vi "ReadParameter.vi"(0 "ParameterConf in":refnum<class "ParameterConf.lvclass">, 3 "error in (no error)":errorcluster, 4 "Parameter":T3(ring)) -> (7 "ParameterConf out":refnum<class "ParameterConf.lvclass">, 8 "DataOut":variant, 9 "DataOutClust":T2, 10 "error out":errorcluster)   [LabVIEW 2014, in "LibraryGcode.lvlib" / "ParameterConf.lvclass"]
uses:
  ParameterConf.lvclass
  control/TypeFirmwareControl.ctl
  ParameterConf.lvclass/ParameterConf.ctl
  LibraryGcode.lvlib
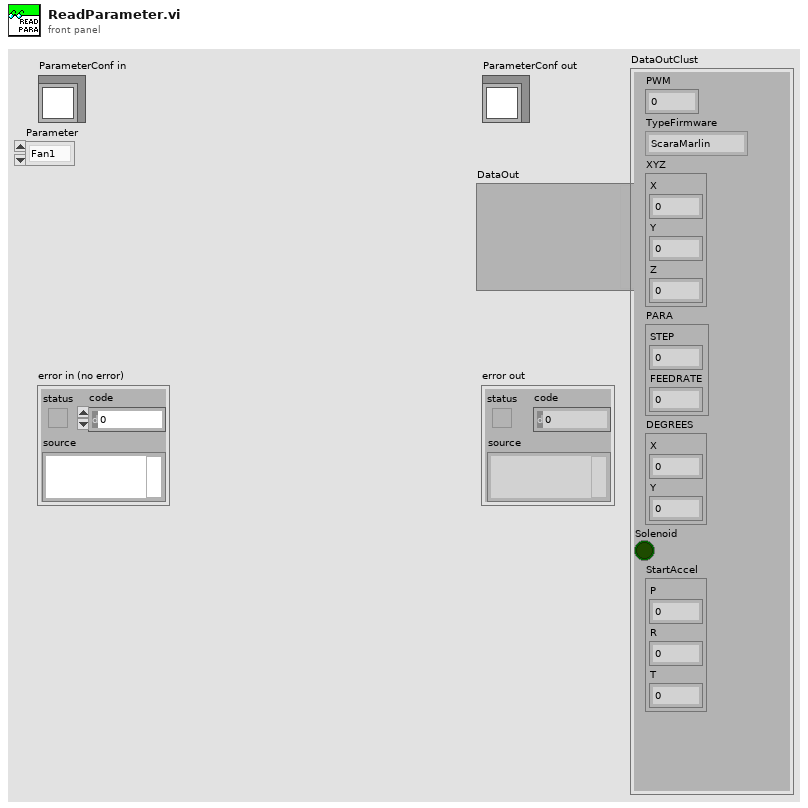
[diagram p1: front panel]
types:
  T1 = typedef "LibraryGcode.lvlib/TypeFirmwareControl.ctl" = enum16{"ScaraMarlin", "CncMarlin", "Mk4Due"}
  T2 = cluster{"PWM":dbl, "TypeFirmware":T1, "XYZ":cluster{"X":dbl, "Y":dbl, "Z":dbl}, "PARA":cluster{"STEP":i16, "FEEDRATE":dbl}, "DEGREES":cluster{"X":dbl, "Y":dbl}, "Solenoid":bool, "StartAccel":cluster{"P":dbl, "R":dbl, "T":dbl}}
  T3 = enum16{"Fan1", "Fan2", "Fan3", "PARA", "POS_DEGREE", "Solenoid", "Spindle", "TypeFirmware", "WaitPin", "MaxAcel", "MaxFeedrate", "MaxSize", "MaxStartAccel"}
  T4 = cluster{"POS":cluster{"X":dbl, "Y":dbl, "Z":dbl}, "DEGREES":cluster{"X":dbl, "Y":dbl}}
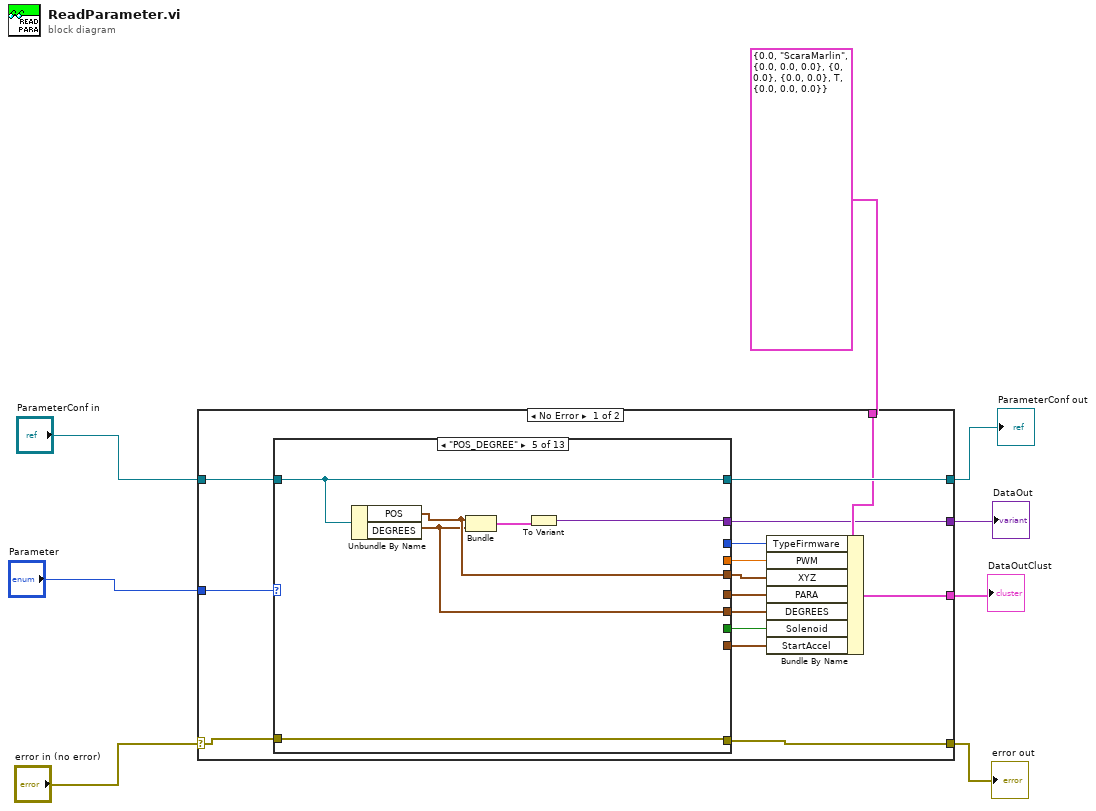
[diagram p0: block diagram]
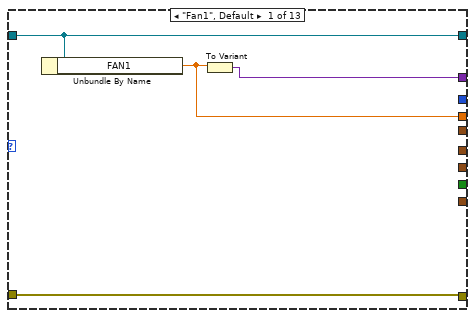
[diagram p2: hidden frame]
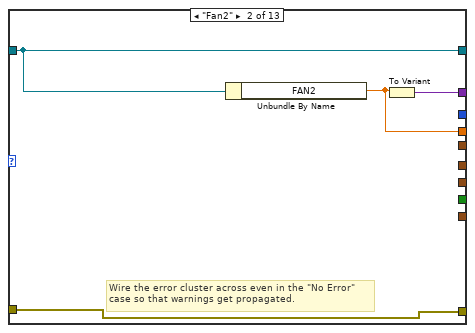
[diagram p3: hidden frame]
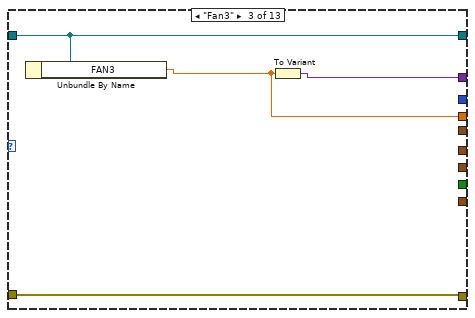
[diagram p4: hidden frame]
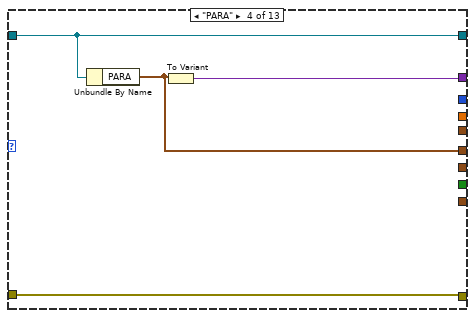
[diagram p5: hidden frame]
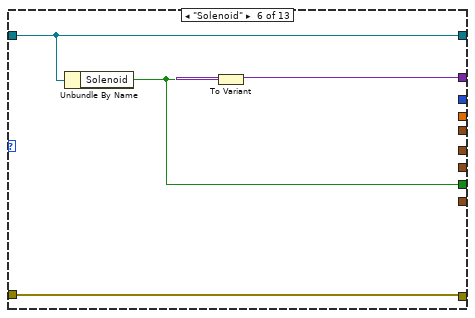
[diagram p6: hidden frame]
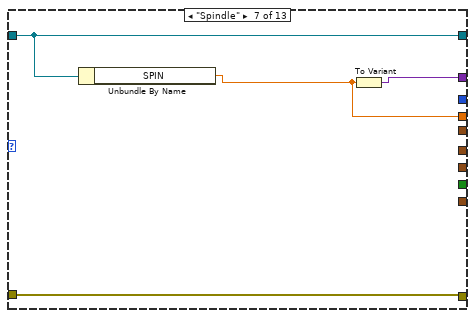
[diagram p7: hidden frame]
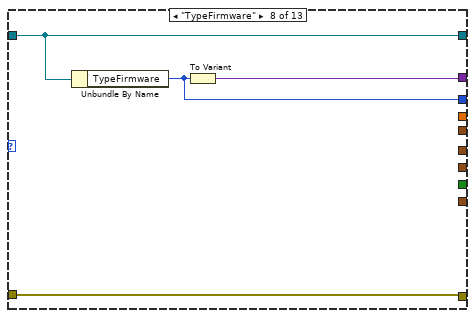
[diagram p8: hidden frame]
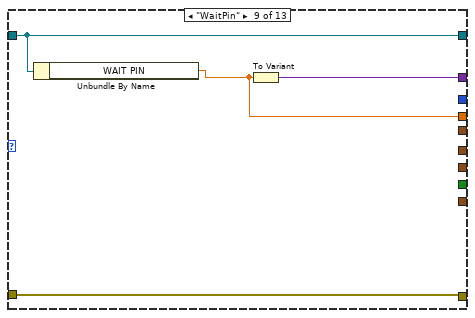
[diagram p9: hidden frame]
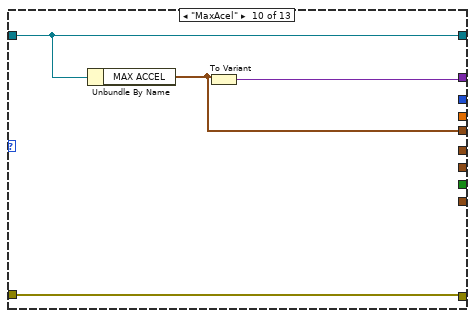
[diagram p10: hidden frame]
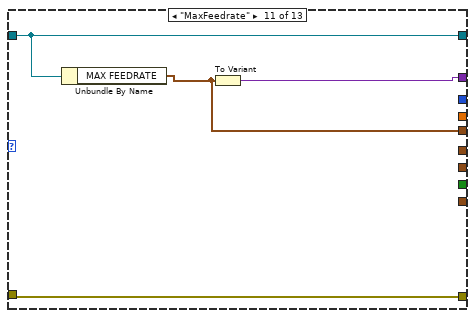
[diagram p11: hidden frame]
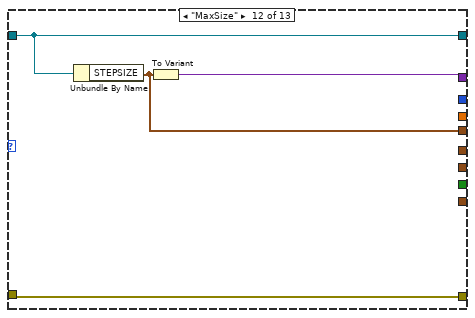
[diagram p12: hidden frame]
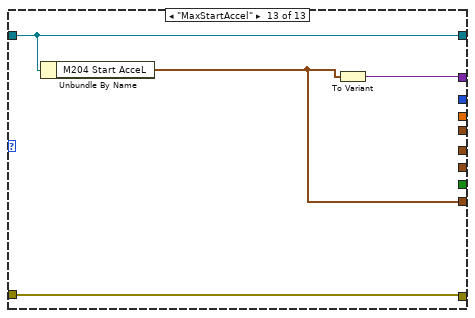
[diagram p13: hidden frame]
diagram:
  n1 = case shown="No Error" "error in (no error)" {
    selector: "error in (no error)" -> [w20 w79]
    tunnel: [w21 w79] -> w7
    tunnel: [w23 w78] -> w5
    tunnel: "ParameterConf in" -> [w22 w78]
    tunnel: "Parameter" -> [w19 _]
    tunnel: [w16 _] -> w3
    tunnel: T2 {"PWM"=0.0, "TypeFirmware"=enum."ScaraMarlin", "XYZ"={"X"=0.0, "Y"=0.0, "Z"=0.0}, "PARA"={"STEP"=0, "FEEDRATE"=0.0}, "DEGREES"={"X"=0.0, "Y"=0.0}, "Solenoid"=TRUE, "StartAccel"={"P"=0.0, "R"=0.0, "T"=0.0}} ("input cluster") -> [w18 _]
    tunnel: [w9 _] -> w1
    frame No Error {
      n2 = case shown="\"POS_DEGREE\"" w19 {
        tunnel: [w27 w30 w35 w39 w45 w49 w53 w57 w60 w64 w69 w73 w76] -> w23
        tunnel: w22 -> [w27 w30 w35 w39 w45 w49 w53 w57 w60 w64 w69 w73 w76]
        tunnel: [w26 w31 w33 w37 w43 w47 w52 w55 w61 w65 w67 w71 w77] -> w21
        tunnel: w20 -> [w26 w31 w33 w37 w43 w47 w52 w55 w61 w65 w67 w71 w77]
        tunnel: [w25 w29 w34 w38 w44 w48 w51 w56 w59 w63 w68 w72 w75] -> w16
        tunnel: [_ _ _ _ w41 _ _ _ _ w62 w66 w70 _] -> w17
        tunnel: [w24 w28 w32 _ _ _ w50 _ w58 _ _ _ _] -> w15
        tunnel: [_ _ _ w36 _ _ _ _ _ _ _ _ _] -> w14
        tunnel: [_ _ _ _ w40 _ _ _ _ _ _ _ _] -> w13
        tunnel: [_ _ _ _ _ w46 _ _ _ _ _ _ _] -> w12
        tunnel: [_ _ _ _ _ _ _ w54 _ _ _ _ _] -> w11
        tunnel: [_ _ _ _ _ _ _ _ _ _ _ _ w74] -> w10
        frame "Fan1", Default {
          n3 = Unbundle By Name(w27) -> ("FAN1"=w24:dbl)
          n4 = To Variant(anything=w24) -> (Variant=w25:variant)
        }
        frame "Fan2" {
          # "Wire the error cluster across even in the \"No Error\"\ncase so that warnings get propagated."
          n5 = Unbundle By Name(w30) -> ("FAN2"=w28:dbl)
          n6 = To Variant(anything=w28) -> (Variant=w29:variant)
        }
        frame "Fan3" {
          n7 = Unbundle By Name(w35) -> ("FAN3"=w32:dbl)
          n8 = To Variant(anything=w32) -> (Variant=w34:variant)
        }
        frame "PARA" {
          n9 = Unbundle By Name(w39) -> ("PARA"=w36:cluster{"STEP":i16, "FEEDRATE":dbl})
          n10 = To Variant(anything=w36) -> (Variant=w38:variant)
        }
        frame "POS_DEGREE" {
          n11 = Unbundle By Name(w45) -> ("POS"=w41:cluster{"X":dbl, "Y":dbl, "Z":dbl}, "DEGREES"=w40:cluster{"X":dbl, "Y":dbl})
          n12 = Bundle("POS"=w41, "DEGREES"=w40) -> (w42:T4)  [unwired: 1 in]
          n13 = To Variant(anything=w42) -> (Variant=w44:variant)
        }
        frame "Solenoid" {
          n14 = Unbundle By Name(w49) -> ("Solenoid"=w46:bool)
          n15 = To Variant(anything=w46) -> (Variant=w48:variant)
        }
        frame "Spindle" {
          n16 = Unbundle By Name(w53) -> ("SPIN"=w50:dbl)
          n17 = To Variant(anything=w50) -> (Variant=w51:variant)
        }
        frame "TypeFirmware" {
          n18 = Unbundle By Name(w57) -> ("TypeFirmware"=w54:T1)
          n19 = To Variant(anything=w54) -> (Variant=w56:variant)
        }
        frame "WaitPin" {
          n20 = Unbundle By Name(w60) -> ("WAIT PIN"=w58:dbl)
          n21 = To Variant(anything=w58) -> (Variant=w59:variant)
        }
        frame "MaxAcel" {
          n22 = Unbundle By Name(w64) -> ("MAX ACCEL"=w62:cluster{"X":dbl, "Y":dbl, "Z":dbl})
          n23 = To Variant(anything=w62) -> (Variant=w63:variant)
        }
        frame "MaxFeedrate" {
          n24 = Unbundle By Name(w69) -> ("MAX FEEDRATE"=w66:cluster{"X":dbl, "Y":dbl, "Z":dbl})
          n25 = To Variant(anything=w66) -> (Variant=w68:variant)
        }
        frame "MaxSize" {
          n26 = Unbundle By Name(w73) -> ("STEPSIZE"=w70:cluster{"X":dbl, "Y":dbl, "Z":dbl})
          n27 = To Variant(anything=w70) -> (Variant=w72:variant)
        }
        frame "MaxStartAccel" {
          n28 = Unbundle By Name(w76) -> ("M204 Start AcceL"=w74:cluster{"P":dbl, "R":dbl, "T":dbl})
          n29 = To Variant(anything=w74) -> (Variant=w75:variant)
        }
      }
      n30 = Bundle By Name(cluster=w18, "TypeFirmware"=w11, "PWM"=w15, "XYZ"=w17, "PARA"=w14, "DEGREES"=w13, "Solenoid"=w12, "StartAccel"=w10) -> (w9:T2)
    }
    frame Error {
    }
  }
  "error out" <- w7
  "ParameterConf out" <- w5
  "DataOut" <- w3
  "DataOutClust" <- w1
